vi "Wavelet Transform Daubechies4 PtByPt.vi"(2 "initialize":bool, 3 "sample length":i32=128, 5 "x":dbl format="%0.2f") -> (0 "error":i32, 1 "Wavelet Daubechies4 {X}":dbl[](array[numeric]))   [LabVIEW 2020, in "NI_PtbyPt.lvlib"]
doc: "Performs the wavelet transform based on the Daubechies4 function."
uses:
  NI_PtbyPt.lvlib
  Real Dot Product.vi
  NI_Gmath.lvlib
  NI_AALBase.lvlib
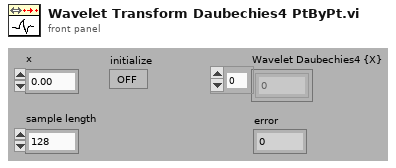
[diagram p1: front panel]
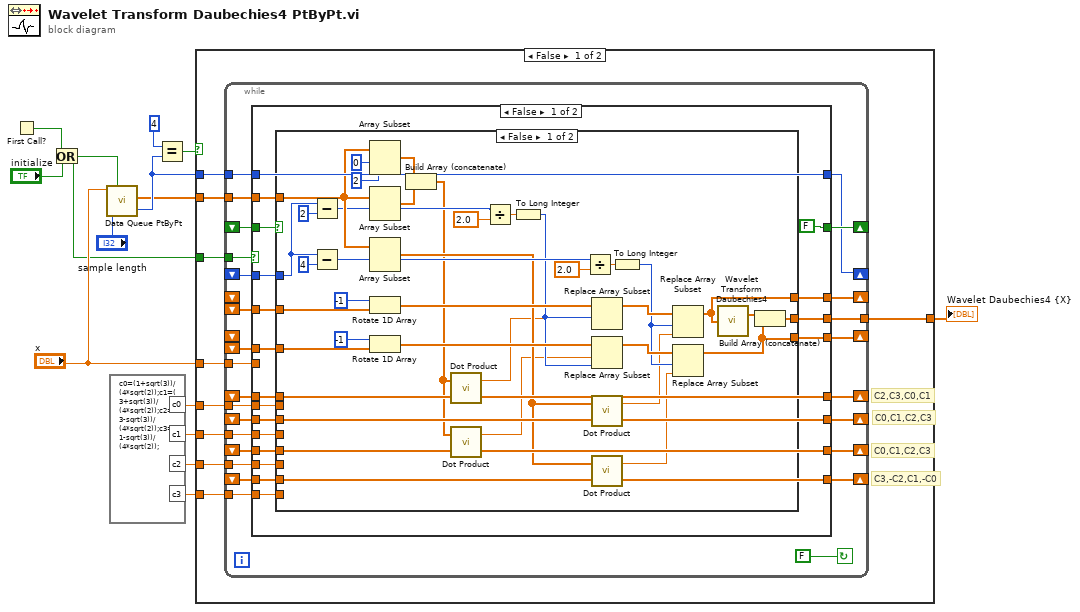
[diagram p0: block diagram]
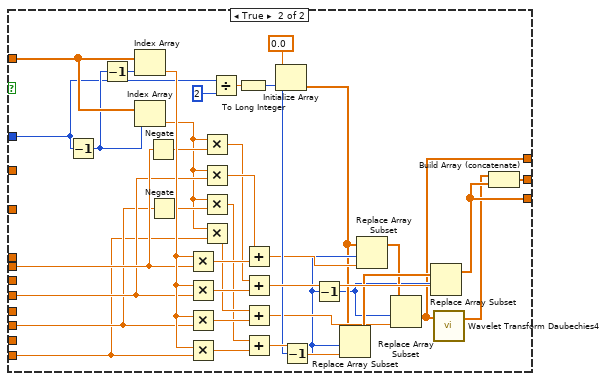
[diagram p2: hidden frame]
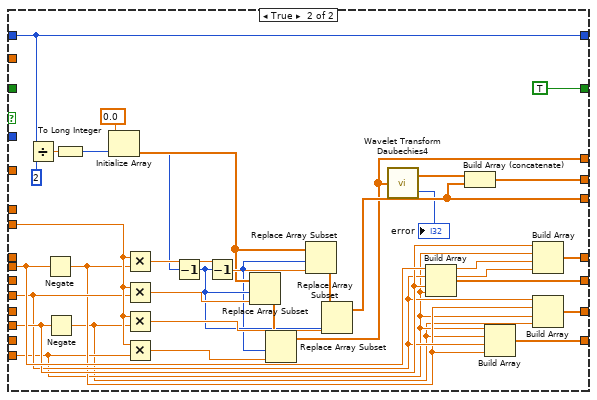
[diagram p3: hidden frame]
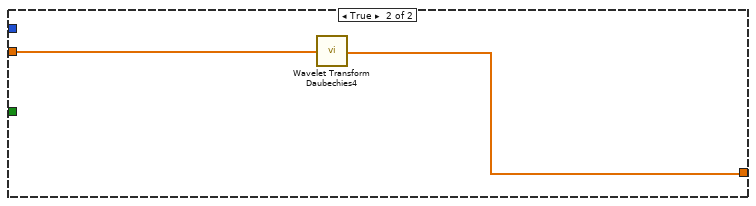
[diagram p4: hidden frame]
diagram:
  n1 = First Call?() -> (First Call?: T/F=w2:bool)
  n2 = Or(x=w2, y="initialize") -> (x .or. y?=w1:bool)
  n3 = call "Data Queue PtByPt.vi"("initialize"=w1, "sample length"="sample length", "input data point"="x") -> ("Current Queue"=w4:dbl[], "current length"=w6:i32)  [unwired: 4 in, 3 out]
  n4 = formula code="c0=(1+sqrt(3))/(4*sqrt(2));c1=(3+sqrt(3))/(4*sqrt(2));c2=(3-sqrt(3))/(4*sqrt(2));c3=(1-sqrt(3))/(4*sqrt(2));"() -> ("c0"=w14:dbl, "c1"=w13:dbl, "c2"=w12:dbl, "c3"=w11:dbl)
  n5 = Equal?(x=4, y=w6) -> (x = y?=w8:bool)
  n6 = case shown="False" w8 {
    tunnel: w1 -> [w23 _]
    tunnel: w14 -> [w22 _]
    tunnel: w13 -> [w21 _]
    tunnel: w12 -> [w20 _]
    tunnel: w11 -> [w19 _]
    tunnel: "x" -> [w18 _]
    tunnel: w4 -> [w17 w175]
    tunnel: [w16 w174] -> w9
    tunnel: w6 -> [w15 _]
    frame False {
      # "C0,C1,C2,C3"
      # "C2,C3,C0,C1"
      # "C3,-C2,C1,-C0"
      # "C0,C1,C2,C3"
      n7 = while {
        tunnel: w15 -> [w27]
        shift-left: _ -> [w25]
        shift-right: [w26] -> _
        shift-left: _ -> [w28]
        shift-right: [w29] -> _
        shift-left: _ -> [w30]
        shift-right: [w31] -> _
        shift-left: _ -> [w32]
        shift-right: [w34] -> _
        shift-left: _ -> [w33]
        shift-right: [w35] -> _
        shift-left: _ -> [w36]
        shift-left: _ -> [w37]
        shift-left: _ -> [_]
        shift-right: [w38] -> _
        shift-left: _ -> [_]
        shift-right: [w39] -> _
        tunnel: [w40] -> w16
        shift-left: _ -> [w41]
        shift-right: [w42] -> _
        tunnel: w17 -> [w43]
        tunnel: w18 -> [w44]
        tunnel: w19 -> [w45]
        tunnel: w20 -> [w46]
        tunnel: w21 -> [w47]
        tunnel: w22 -> [w48]
        tunnel: w23 -> [w49]
        stop <- FALSE continue-if-true
        n8 = case shown="False" w49 {
          tunnel: w25 -> [w66 _]
          tunnel: w48 -> [w65 w156]
          tunnel: w47 -> [w64 w149]
          tunnel: w46 -> [w63 w151]
          tunnel: w45 -> [w62 w147]
          tunnel: w44 -> [_ w170]
          tunnel: [w61 w161] -> w40
          tunnel: w43 -> [w67 _]
          tunnel: [FALSE TRUE] -> w42
          tunnel: w41 -> [w60 _]
          tunnel: [w59 w152] -> w39
          tunnel: [w58 w157] -> w38
          tunnel: w37 -> [w57 _]
          tunnel: w36 -> [w56 _]
          tunnel: [w55 w155] -> w35
          tunnel: [w54 w154] -> w34
          tunnel: w33 -> [w55 _]
          tunnel: w32 -> [w54 _]
          tunnel: [w52 w150] -> w31
          tunnel: w30 -> [w52 _]
          tunnel: [w53 w145] -> w29
          tunnel: w28 -> [w53 _]
          tunnel: [w51 w144] -> w26
          tunnel: w27 -> [w51 w144]
          frame False {
            n9 = case shown="False" w60 {
              tunnel: w67 -> [w98 w142]
              tunnel: w66 -> [w97 w118]
              tunnel: w65 -> [_ w137]
              tunnel: w64 -> [_ w136]
              tunnel: w63 -> [_ w135]
              tunnel: w62 -> [_ w134]
              tunnel: [w84 w109] -> w61
              tunnel: [w83 w106] -> w59
              tunnel: [w82 w108] -> w58
              tunnel: w57 -> [w105 _]
              tunnel: w56 -> [w104 _]
              tunnel: w55 -> [w79 _]
              tunnel: w54 -> [w78 _]
              tunnel: w53 -> [w71 _]
              tunnel: w52 -> [w72 _]
              frame False {
                n10 = Subtract(x=w97, y=2) -> (x-y=w90:i32)
                n11 = Subtract(x=w97, y=4) -> (x-y=w88:i32)
                n12 = Array Subset(array=w98, index=0 ("Array Index"), length=2 ("Array Length")) -> (w81:dbl[])
                n13 = Array Subset(array=w98, index=w90) -> (w80:dbl[])  [unwired: 1 in]
                n14 = Array Subset(array=w98, index=w88) -> (w77:dbl[])  [unwired: 1 in]
                n15 = Rotate 1D Array(1:w105, 2:i16 -1 ("n")) -> (0:w95:dbl[])
                n16 = Rotate 1D Array(1:w104, 2:i16 -1 ("n")) -> (0:w94:dbl[])
                n17 = Build Array (concatenate)(w81, w80) -> (w70:dbl[])
                n18 = call-poly "Dot Product.vi"("Y Vector"=w72, "X Vector"=w70) -> ("X * Y"=w69:dbl)  [unwired: 1 out]
                n19 = call-poly "Dot Product.vi"("Y Vector"=w71, "X Vector"=w70) -> ("X * Y"=w68:dbl)  [unwired: 1 out]
                n20 = Divide(x=w90, y=2.0) -> (x/y=w87:dbl)
                n21 = To Long Integer(number=w87) -> (32bit integer=w75:i32)
                n22 = Divide(x=w88, y=2.0) -> (x/y=w86:dbl)
                n23 = Replace Array Subset(array=w95, new element=w69, index=w75) -> (w93:dbl[])
                n24 = Replace Array Subset(array=w94, new element=w68, index=w75) -> (w92:dbl[])
                n25 = call-poly "Dot Product.vi"("Y Vector"=w79, "X Vector"=w77) -> ("X * Y"=w74:dbl)  [unwired: 1 out]
                n26 = call-poly "Dot Product.vi"("Y Vector"=w78, "X Vector"=w77) -> ("X * Y"=w73:dbl)  [unwired: 1 out]
                n27 = To Long Integer(number=w86) -> (32bit integer=w76:i32)
                n28 = Replace Array Subset(array=w93, new element=w74, index=w76) -> (w83:dbl[])
                n29 = Replace Array Subset(array=w92, new element=w73, index=w76) -> (w82:dbl[])
                n30 = call "Wavelet Transform Daubechies4.vi"("X"=w83) -> ("Wavelet Daubechies4 {X}"=w85:dbl[])  [unwired: 1 out]
                n31 = Build Array (concatenate)(w85, w82) -> (w84:dbl[])
              }
              frame True {
                n32 = Decrement(x=w118) -> (x-1=w141:i32)
                n33 = Decrement(x=w141) -> (x-1=w119:i32)
                n34 = Index Array(array=w142, index=w119) -> (element=w140:dbl)
                n35 = Index Array(array=w142, index=w141) -> (element=w133:dbl)
                n36 = Negate(x=w137) -> (-x=w139:dbl)
                n37 = Negate(x=w135) -> (-x=w138:dbl)
                n38 = Multiply(x=w140, y=w137) -> (x*y=w129:dbl)
                n39 = Multiply(x=w140, y=w136) -> (x*y=w130:dbl)
                n40 = Multiply(x=w140, y=w135) -> (x*y=w131:dbl)
                n41 = Multiply(x=w140, y=w134) -> (x*y=w132:dbl)
                n42 = Multiply(x=w133, y=w139) -> (x*y=w127:dbl)
                n43 = Multiply(x=w133, y=w136) -> (x*y=w128:dbl)
                n44 = Multiply(x=w133, y=w138) -> (x*y=w125:dbl)
                n45 = Multiply(x=w133, y=w134) -> (x*y=w126:dbl)
                n46 = Divide(x=w118, y=2) -> (x/y=w123:dbl)
                n47 = To Long Integer(number=w123) -> (32bit integer=w117:i32)
                n48 = Add(x=w128, y=w129) -> (x+y=w114:dbl)
                n49 = Add(x=w127, y=w130) -> (x+y=w120:dbl)
                n50 = Add(x=w126, y=w131) -> (x+y=w115:dbl)
                n51 = Add(x=w125, y=w132) -> (x+y=w121:dbl)
                n52 = Initialize Array(0.0 ("Element Data"), w117) -> (w112:dbl[])
                n53 = Decrement(x=w117) -> (x-1=w113:i32)
                n54 = Decrement(x=w113) -> (x-1=w110:i32)
                n55 = Replace Array Subset(array=w112, new element=w121, index=w113) -> (w116:dbl[])
                n56 = Replace Array Subset(array=w112, new element=w114, index=w113) -> (w111:dbl[])
                n57 = Replace Array Subset(array=w111, new element=w115, index=w110) -> (w106:dbl[])
                n58 = Replace Array Subset(array=w116, new element=w120, index=w110) -> (w108:dbl[])
                n59 = call "Wavelet Transform Daubechies4.vi"("X"=w106) -> ("Wavelet Daubechies4 {X}"=w107:dbl[])  [unwired: 1 out]
                n60 = Build Array (concatenate)(w107, w108) -> (w109:dbl[])
              }
            }
          }
          frame True {
            n61 = Divide(x=w144, y=2) -> (x/y=w172:dbl)
            n62 = Negate(x=w156) -> (-x=w148:dbl)
            n63 = Negate(x=w151) -> (-x=w146:dbl)
            n64 = To Long Integer(number=w172) -> (32bit integer=w163:i32)
            n65 = Initialize Array(0.0 ("Element Data"), w163) -> (w164:dbl[])
            n66 = Multiply(x=w170, y=w148) -> (x*y=w166:dbl)
            n67 = Multiply(x=w170, y=w149) -> (x*y=w167:dbl)
            n68 = Multiply(x=w170, y=w146) -> (x*y=w168:dbl)
            n69 = Multiply(x=w170, y=w147) -> (x*y=w169:dbl)
            n70 = Decrement(x=w163) -> (x-1=w160:i32)
            n71 = Decrement(x=w160) -> (x-1=w159:i32)
            n72 = Replace Array Subset(array=w164, new element=w167, index=w160) -> (w162:dbl[])
            n73 = Replace Array Subset(array=w162, new element=w169, index=w159) -> (w152:dbl[])
            n74 = Replace Array Subset(array=w164, new element=w166, index=w159) -> (w165:dbl[])
            n75 = Replace Array Subset(array=w165, new element=w168, index=w160) -> (w157:dbl[])
            n76 = call "Wavelet Transform Daubechies4.vi"("X"=w152) -> ("Wavelet Daubechies4 {X}"=w153:dbl[], "error"=→"error":i32)
            n77 = Build Array(w156, w149, w151, w147) -> (w155:dbl[])
            n78 = Build Array (concatenate)(w153, w157) -> (w161:dbl[])
            n79 = Build Array(w147, w146, w149, w148) -> (w154:dbl[])
            n80 = Build Array(w151, w147, w156, w149) -> (w150:dbl[])
            n81 = Build Array(w149, w148, w147, w146) -> (w145:dbl[])
          }
        }
      }
    }
    frame True {
      n82 = call "Wavelet Transform Daubechies4.vi"("X"=w175) -> ("Wavelet Daubechies4 {X}"=w174:dbl[])  [unwired: 1 out]
    }
  }
  "Wavelet Daubechies4 {X}" <- w9
